vi "Result To Error.vi"(8 "error in (no error)":errorcluster, 11 "Result Code":i32) -> (0 "error out":errorcluster)   [LabVIEW 2020, in "G-Image.lvlib"]
doc: "Converts the result codes found in g_image.h to a custom LabVIEW error code. The custom error code range begins at 559513."
uses:
  G-Image.lvlib
  <vilib>/Utility/error.llb/Error Cluster From Error Code.vi
  <vilib>/ErrorRing/Error Ring.xnode
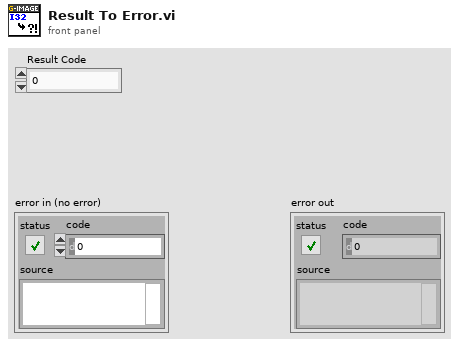
[diagram p1: front panel]
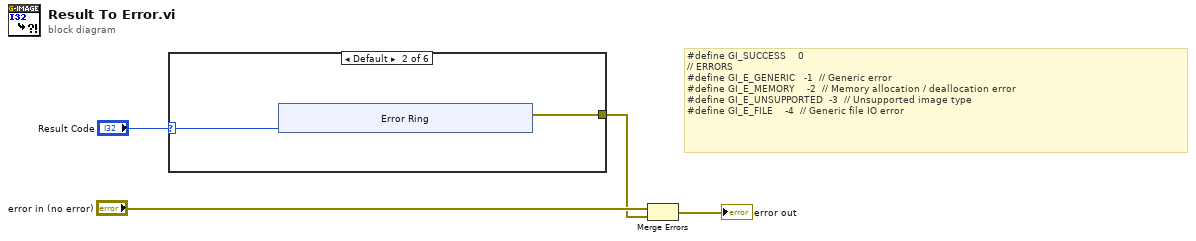
[diagram p0: block diagram]
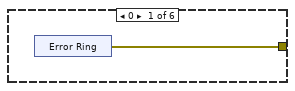
[diagram p2: hidden frame]
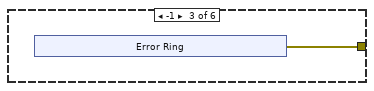
[diagram p3: hidden frame]
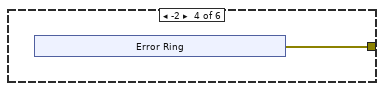
[diagram p4: hidden frame]
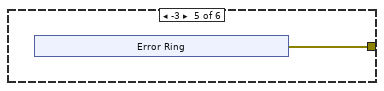
[diagram p5: hidden frame]
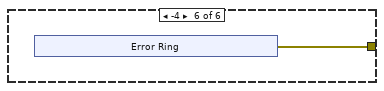
[diagram p6: hidden frame]
diagram:
  # "#define GI_SUCCESS\t\t\t\t0\n// ERRORS\n#define GI_E_GENERIC\t\t\t-1\t\t// Generic error\n#define GI_E_MEMORY\t\t\t\t-2\t\t// Memory allocation / deallocation error\n#define GI_E_UNSUPPORTED\t\t-3\t\t// Unsupported image type\n#define GI_E_FILE\t\t\t\t-4\t\t// Generic file IO error"
  n1 = case shown="Default" "Result Code" {
    selector: "Result Code" -> [_ w7 _ _ _ _]
    tunnel: [w5 w8 w16 w22 w28 w34] -> w1
    frame 0 {
      n2 = xnode "Error Ring"() -> ("error out"=w5:errorcluster)
    }
    frame Default {
      n3 = xnode "Error Ring"("parameter 0"=w7) -> ("error out"=w8:errorcluster)
    }
    frame -1 {
      n4 = xnode "Error Ring"() -> ("error out"=w16:errorcluster)
    }
    frame -2 {
      n5 = xnode "Error Ring"() -> ("error out"=w22:errorcluster)
    }
    frame -3 {
      n6 = xnode "Error Ring"() -> ("error out"=w28:errorcluster)
    }
    frame -4 {
      n7 = xnode "Error Ring"() -> ("error out"=w34:errorcluster)
    }
  }
  n8 = Merge Errors("error in (no error)", w1) -> (→"error out":errorcluster)
